vi "Select Option.vi"(8 "error in":errorcluster) -> (0 "error out":errorcluster, 2 "String Value":string)   [LabVIEW 2018]
uses:
  <vilib>/Utility/file.llb/Read Delimited Spreadsheet (string).vi
panel:
  in  "OK Button":bool
  in  "Numeric Control":string(combo)
  # "Select the Tester Function"
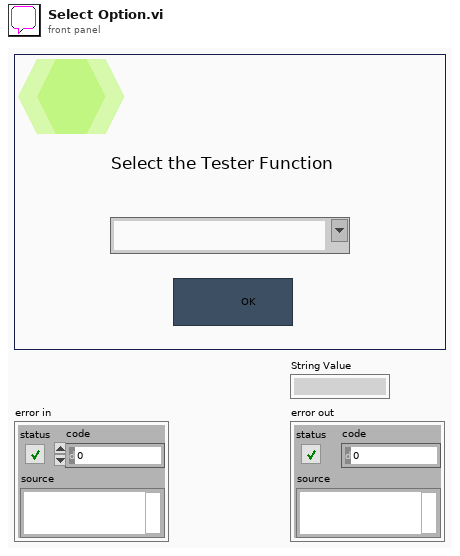
[diagram p1: front panel]
types:
  T1 = enum32{"invalid app kind", "Development System", "Run Time System", "Student Edition", "Embedded LabVIEW", "Evaluation", "Custom"}
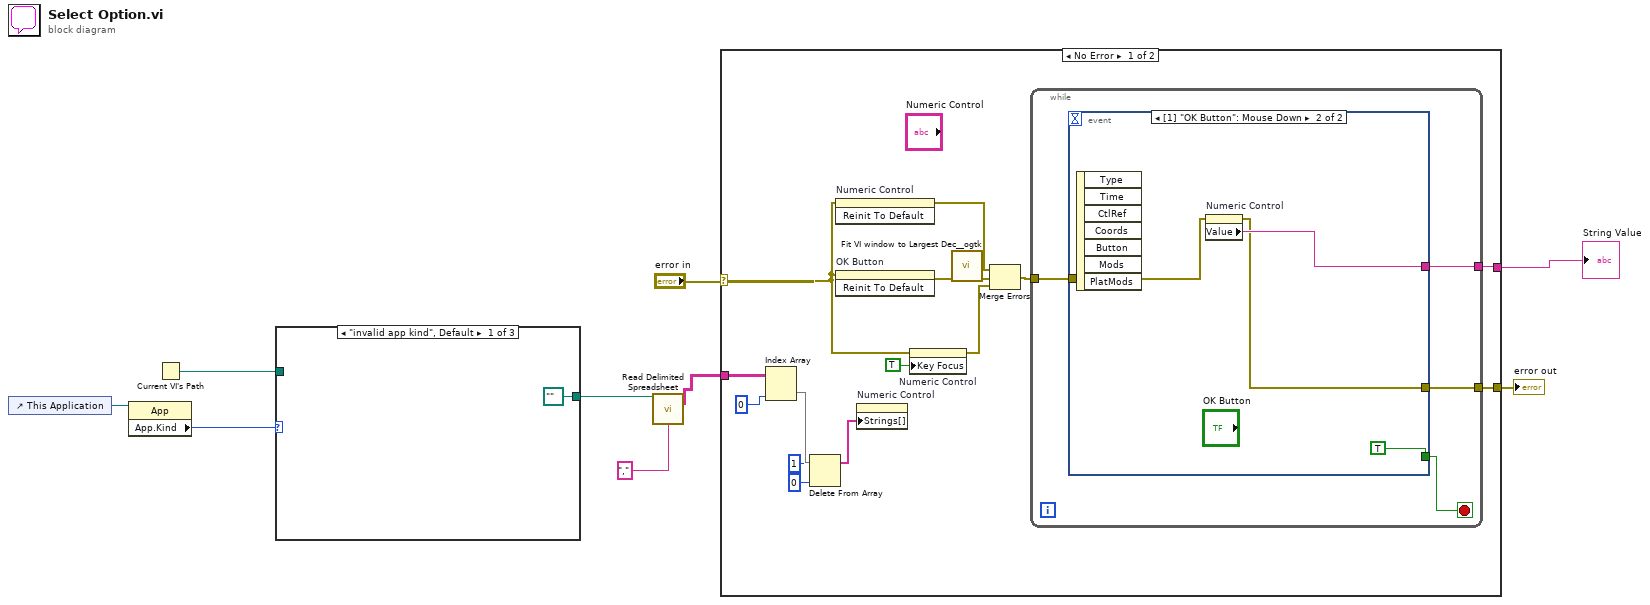
[diagram p0: block diagram]
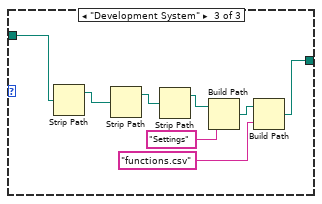
[diagram p3: hidden frame]
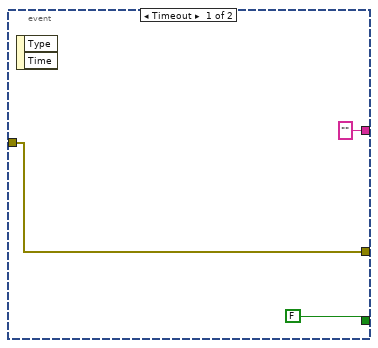
[diagram p4: hidden frame]
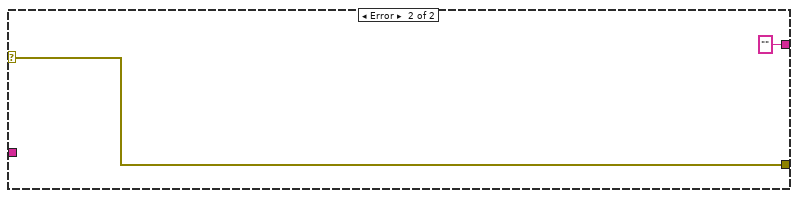
[diagram p5: hidden frame]
diagram:
  n1 = control-ref of="This Application"() -> (w6:refnum<vi>)
  n2 = property class="App"(reference=w6) -> ("App.Kind"=w5:T1)  [unwired: 1 in, 2 out]
  n3 = Current VI's Path() -> (path=w4:path)
  n4 = case shown="\"invalid app kind\", Default" w5 {
    tunnel: w4 -> [_ w11 w13]
    tunnel: [path "" ("appended path") w11 w14] -> w3
    frame "invalid app kind", Default {
    }
    frame "Run Time System" {
    }
    frame "Development System" {
      n5 = Strip Path(path=w13) -> (stripped path=w12:path)  [unwired: 1 out]
      n6 = Strip Path(path=w12) -> (stripped path=w19:path)  [unwired: 1 out]
      n7 = Strip Path(path=w19) -> (stripped path=w18:path)  [unwired: 1 out]
      n8 = Build Path(base path=w18, name or relative path="Settings") -> (appended path=w16:path)
      n9 = Build Path(base path=w16, name or relative path="functions.csv") -> (appended path=w14:path)
    }
  }
  n10 = call-poly <vilib>:"Read Delimited Spreadsheet.vi"("file path (dialog if empty)"=w3, "delimiter (\\t)"="," ("delimiter (\\t)")) -> ("all rows"=w1:string[][])  [unwired: 8 in, 5 out]
  n11 = case shown="No Error" "error in" {
    selector: "error in" -> [w20 w47]
    tunnel: [w33 "" ("Value")] -> w9
    tunnel: [w32 w47] -> w7
    tunnel: w1 -> [w27 _]
    frame No Error {
      n12 = Index Array(array=w27, index (col)=0 ("index")) -> (element=w25:string[])  [unwired: 1 in]
      n13 = Delete From Array(array=w25, length=1, index=0) -> (array with subset deleted=w24:string[])  [unwired: 1 out]
      n14 = invoke on="Numeric Control" class="CmbBox" method="Reinit To Default"(error in=w20) -> (error out=w21:errorcluster)  [unwired: 2 in, 2 out]
      n15 = invoke on="OK Button" class="Bool" method="Reinit To Default"(error in=w20) -> (error out=w34:errorcluster)  [unwired: 2 in, 2 out]
      n16 = property on="Numeric Control" class="CmbBox"("Strings[]"=w24) -> ()  [unwired: 2 in, 2 out]
      n17 = property on="Numeric Control" class="CmbBox"(error in=w20, "Key Focus"=TRUE) -> (error out=w29:errorcluster)  [unwired: 1 in, 1 out]
      n18 = call <userlib>:"Fit VI window to Largest Dec__ogtk.vi"("error in (no error)"=w34) -> ("error out"=w30:errorcluster)  [unwired: 5 in, 1 out]
      n19 = Merge Errors(w21, w30, w29) -> (w28:errorcluster)
      n20 = while {
        tunnel: w28 -> [w38]
        tunnel: [w37] -> w33
        tunnel: [w36] -> w32
        stop <- w35 stop-if-true
        n21 = event shown="[1] \"OK Button\": Mouse Down" {
          selector: _ -> [_ _]
          dyn-events: _ -> [_ _]
          timeout: _ -> [_ _]
          tunnel: w38 -> [w41 w43]
          tunnel: ["" ("Value") w44] -> w37
          tunnel: [w41 w42] -> w36
          tunnel: [FALSE TRUE] -> w35
          event Timeout {
            n22 = event-data() -> ()  [unwired: 1 in, 2 out]
          }
          event "OK Button": Mouse Down {
            n23 = event-data() -> ()  [unwired: 1 in, 7 out]
            n24 = property on="Numeric Control" class="CmbBox"(error in=w43) -> (error out=w42:errorcluster, "Value"=w44:string)  [unwired: 1 in, 1 out]
          }
        }
      }
    }
    frame Error {
    }
  }
  "String Value" <- w9
  "error out" <- w7
